vi "Write Report.vi"(8 "error in (no error)":errorcluster, 10 "Resource In":variant, 11 "Analyze Parameter Fluence in":refnum<class "Analyze Parameter Fluence.lvclass">) -> (0 "error out":errorcluster, 2 "Resource Out":variant, 3 "Analyze Parameter Fluence out":refnum<class "Analyze Parameter Fluence.lvclass">)   [LabVIEW 2020, in "Analyze Parameter Fluence.lvclass"]
uses:
  Analyze Parameter Fluence.lvclass
  C:/POLARIS Programme/POLARIS-AS-3-Cams/Submodules/HIJ Vision/Analyze/Analyze Parameter/Analyze Parameter Base/Analyze Parameter Base.lvclass
  <vilib>/Utility/config.llb/Config Data RefNum.ctl
  Analyze Parameter Fluence.lvclass/Analyze Parameter Fluence.ctl
  <vilib>/Utility/config.llb/Write Key (I32).vi
  Analyze Parameter Base/Analyze Parameter Base.lvclass
  <vilib>/Utility/config.llb/NI_LVConfig.lvlib
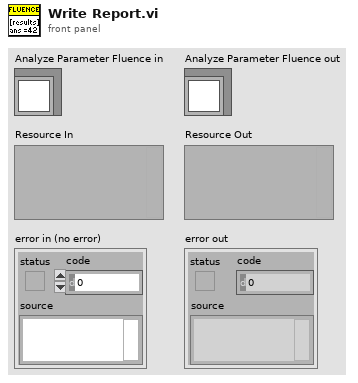
[diagram p1: front panel]
types:
  T1 = typedef "NI_LVConfig.lvlib/Config Data RefNum.ctl" = refnum<k1>
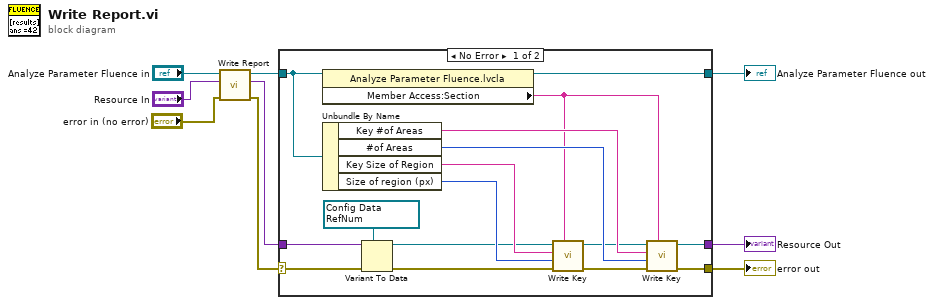
[diagram p0: block diagram]
diagram:
  n1 = call-parent "Write Report.vi"("error in (no error)"="error in (no error)", "Resource In"="Resource In", "Analyze Parameter Base in"="Analyze Parameter Fluence in") -> ("error out"=w5:errorcluster, "Resource Out"=w4:variant, "Analyze Parameter Base out"=w6:refnum<class "Analyze Parameter Fluence.lvclass">)  [unwired: 6 in]
  n2 = case shown="No Error" w5 {
    selector: w5 -> [w15 w28]
    tunnel: w4 -> [w24 w26]
    tunnel: w6 -> [w23 w27]
    tunnel: [w13 w27] -> w1
    tunnel: [w19 w26] -> w3
    tunnel: [w17 w28] -> w2
    frame No Error {
      w16 = T1 refnum items=["config data"] ("refnum")
      n3 = property class="Analyze Parameter Fluence.lvcla"(reference=w23) -> (reference out=w13:refnum<class "Analyze Parameter Fluence.lvclass">, "Member Access:Section"=w21:string)  [unwired: 1 in, 1 out]
      n4 = Unbundle By Name(w23) -> ("Key #of Areas"=w22:string, "#of Areas"=w25:i32, "Key Size of Region"=w12:string, "Size of region (px)"=w11:i32)
      n5 = Variant To Data(error in=w15, type=w16, Variant=w24) -> (data=w10:T1, error out=w14:errorcluster)
      n6 = call-poly <vilib>:"Write Key.vi"("section"=w21, "error in (no error)"=w14, "value"=w11, "key"=w12, "refnum"=w10) -> ("error out"=w18:errorcluster, "refnum out"=w20:T1)  [unwired: 4 in, 1 out]
      n7 = call-poly <vilib>:"Write Key.vi"("section"=w21, "error in (no error)"=w18, "value"=w25, "key"=w22, "refnum"=w20) -> ("error out"=w17:errorcluster, "refnum out"=w19:T1)  [unwired: 4 in, 1 out]
    }
    frame Error {
    }
  }
  "error out" <- w2
  "Analyze Parameter Fluence out" <- w1
  "Resource Out" <- w3
